vi "Verison Cluster to String.vi"(11 "version":T1) -> (3 "version string":string)   [LabVIEW 2021, in "DSF Core.lvlib"]
uses:
  DSF Core.lvlib
  Typedefs/DSF Version Info.ctl
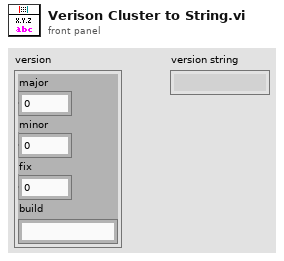
[diagram p1: front panel]
types:
  T1 = typedef "DSF Core.lvlib/DSF Version Info.ctl" = cluster{"major":u32, "minor":u32, "fix":u32, "build":string}
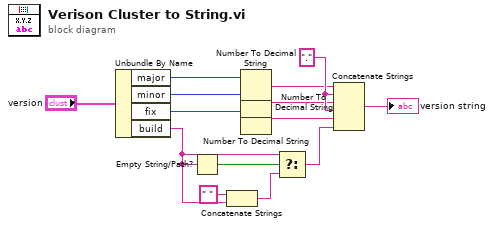
[diagram p0: block diagram]
diagram:
  w10 = "."
  n1 = Unbundle By Name("version") -> ("major"=w13:u32, "minor"=w12:u32, "fix"=w11:u32, "build"=w3:string)
  n2 = Empty String/Path?(string/path=w3) -> (empty?=w5:bool)
  n3 = Concatenate Strings(" " ("string"), w3) -> (w2:string)
  n4 = Number To Decimal String(number=w13) -> (decimal integer string=w7:string)  [unwired: 1 in]
  n5 = Number To Decimal String(number=w12) -> (decimal integer string=w9:string)  [unwired: 1 in]
  n6 = Number To Decimal String(number=w11) -> (decimal integer string=w8:string)  [unwired: 1 in]
  n7 = Select(t=w3, s=w5, f=w2) -> (s? t:f=w1:string)
  n8 = Concatenate Strings(w7, w10, w9, w10, w8, w1) -> (→"version string":string)
